vi "Discard Samples - Filter Delay.vi"(0 "DAQ TSM in":T1, 11 "error in":errorcluster) -> (4 "DAQ TSM Out":T1, 15 "error out":errorcluster)   [LabVIEW 2020]
doc: "Reads one or more waveforms from a task that contains one or more analog input channels. The data will be ordered based on the SSC order."
uses:
  Instrument Control/DAQmx/Pin Map/TSM DAQmx Multi-Task.ctl
  <vilib>/NI_TestStand_SemiconductorModule/NI_TestStand_Semiconductor_Module.lvlibp/PinMap/PinQueryContext/MultiplePinMultipleSessionQueryContext/MultiplePinMultipleSessionQueryContext.lvclass
  Instrument Control/DAQmx/Pin Map/SSC DAQmx.ctl
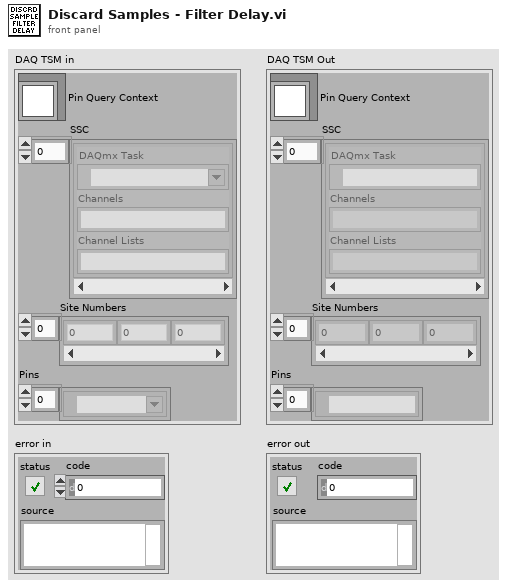
[diagram p1: front panel]
types:
  T1 = typedef "TSM DAQmx Multi-Task.ctl" = cluster{"Pin Query Context":refnum<class "MultiplePinMultipleSessionQueryContext.lvclass">, "SSC":T2[], "Site Numbers":i32[], "Pins":tag[]}
  T2 = typedef "SSC DAQmx.ctl" = cluster{"DAQmx Task ":refnum<k21>, "Channels":string, "Channel Lists":string}
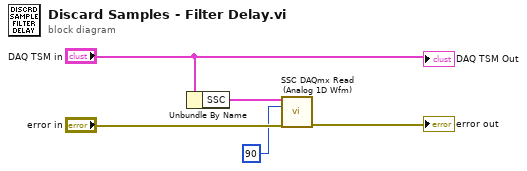
[diagram p0: block diagram]
diagram:
  n1 = Unbundle By Name("DAQ TSM in") -> ("SSC"=w2:T2[])
  n2 = call "SSC DAQmx Read (Analog 1D Wfm).vi"("DAQmx SSC in"=w2, "Samples to read"=90, "error in"="error in") -> ("error out"=→"error out":errorcluster)  [unwired: 10 in, 2 out]
  "DAQ TSM Out" <- "DAQ TSM in"
